vi "recalibrate magnetometers from h5.vi"(0 "file":string, 1 "calibrated_data":dbl, 5 "local_field_magnitude":dbl, 7 "calibration_block":string, 9 "uncalibrated_data":dbl, 12 "num_samples":i32) -> (3 "calibrated_data out":dbl, 4 "file out":string, 6 "function return":i32, 8 "calibration_block out":string, 10 "uncalibrated_data out":dbl, 14 "num_samples out":i32)   [LabVIEW 2019, in "apdm.lvlib"]
doc: "APDM_EXPORT int apdm_recalibrate_magnetometers_from_h5(char *file, double local_field_magnitude, uint8_t *calibration_block, double *uncalibrated_data, double *calibrated_data, int32_t *num_samples);"
uses:
  apdm.lvlib
  Lee Lab/CP FES Walking 2018/Code/Working/LabVIEW/apdm.dll
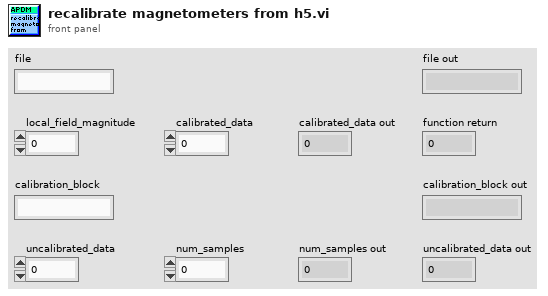
[diagram p1: front panel]
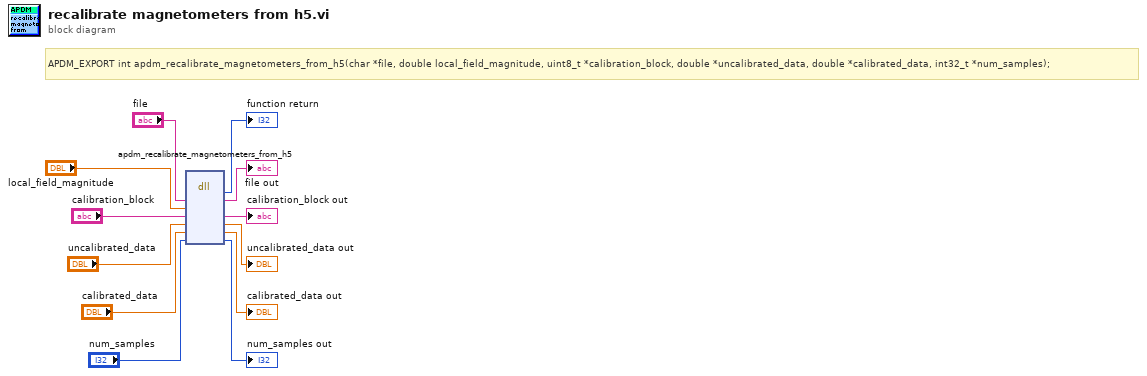
[diagram p0: block diagram]
diagram:
  # "APDM_EXPORT int apdm_recalibrate_magnetometers_from_h5(char *file, double local_field_magnitude, uint8_t *calibration_block, double *uncalibrated_data, double *calibrated_data, int32_t *num_samples);"
  n1 = dll-call lib="C:/Users/jfalesi/Dropbox/Lee Lab/CP FES Walking 2018/Code/Working/LabVIEW/apdm.*" fn="apdm_recalibrate_magnetometers_from_h5"("file"="file", "local_field_magnitude"="local_field_magnitude", "calibration_block"="calibration_block", "uncalibrated_data"="uncalibrated_data", "calibrated_data"="calibrated_data", "num_samples"="num_samples") -> (→"function return":i32, "file"=→"file out":string, "calibration_block"=→"calibration_block out":string, "uncalibrated_data"=→"uncalibrated_data out":dbl, "calibrated_data"=→"calibrated_data out":dbl, "num_samples"=→"num_samples out":i32)  [unwired: 4 in, 2 out]
